vi "Create Polygon List.vi"(8 "error in (no error)":errorcluster) -> (0 "error out":errorcluster, 3 "specific class reference":refnum<k24>)   [LabVIEW 2014]
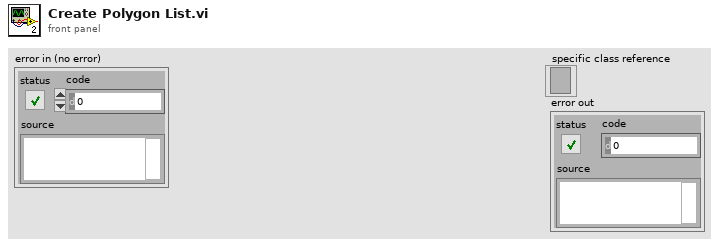
[diagram p1: front panel]
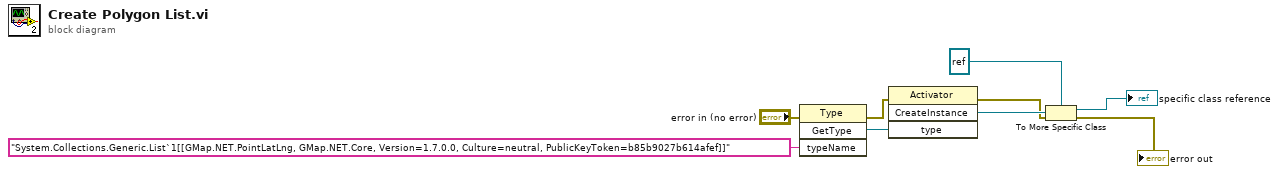
[diagram p0: block diagram]
diagram:
  n1 = invoke class="Type" method="GetType"(error in="error in (no error)", "typeName"="System.Collections.Generic.List`1[[GMap.NET.PointLatLng, GMap.NET.Core, Version=1.7.0.0, Culture=neutral, PublicKeyToken=b85b9027b614afef]]") -> (error out=w2:errorcluster, "GetType"=w8:refnum<k24>)  [unwired: 2 in, 2 out]
  n2 = invoke class="Activator" method="CreateInstance"(error in=w2, "type"=w8) -> (error out=w6:errorcluster, "CreateInstance"=w7:refnum<k24>)  [unwired: 2 in, 2 out]
  n3 = To More Specific Class(target class=refnum<k24> refnum ("points"), reference=w7, error in=w6) -> (specific class reference=→"specific class reference":refnum<k24>, error out=→"error out":errorcluster)
